vi "ConvertDataDoubleToDriveStatus.vi"(8 "error in (no error)":errorcluster, 9 "Drive Status":string(combo)="MaskValue", 10 "Double In":dbl[](array[numeric]), 11 "controller in":refnum<k24>) -> (0 "error out":errorcluster, 2 "Drive Status Out":i32[](array[numeric]), 3 "controller out":refnum<k24>)   [LabVIEW 2010]
uses:
  c:/aerotech/controller/dev/A3200/pc/labview/2010/bin/Aerotech.A3200.dll
  bin/Aerotech.A3200.dll
  c:/aerotech/controller/dev/A3200/pc/labview/2010/bin/Aerotech.A3200.LabVIEW.dll
  bin/Aerotech.A3200.LabVIEW.dll
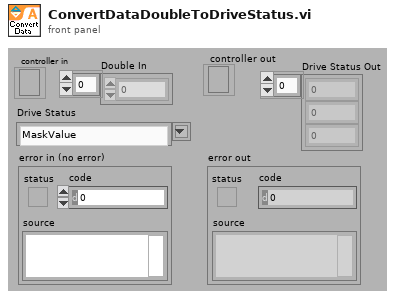
[diagram p1: front panel]
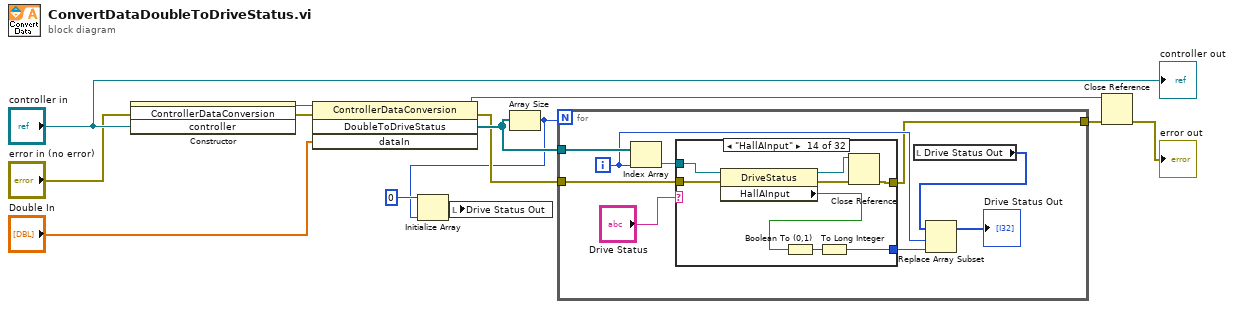
[diagram p0: block diagram]
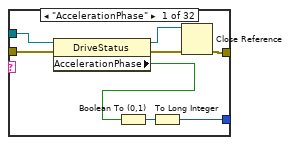
[diagram p2: hidden frame]
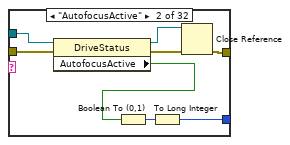
[diagram p3: hidden frame]
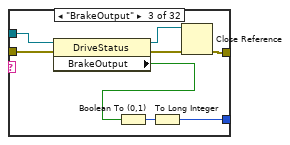
[diagram p4: hidden frame]
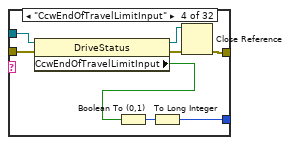
[diagram p5: hidden frame]
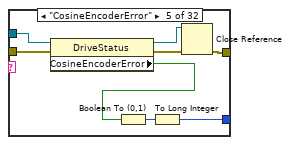
[diagram p6: hidden frame]
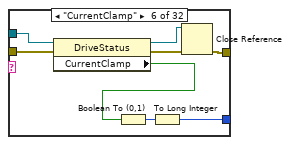
[diagram p7: hidden frame]
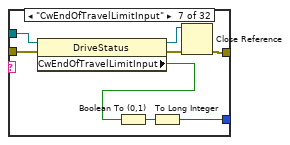
[diagram p8: hidden frame]
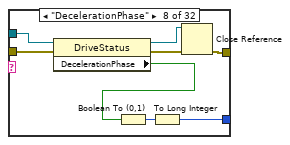
[diagram p9: hidden frame]
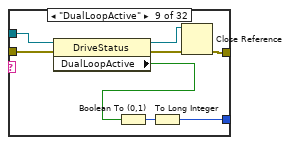
[diagram p10: hidden frame]
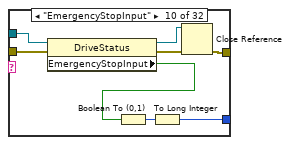
[diagram p11: hidden frame]
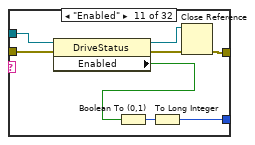
[diagram p12: hidden frame]
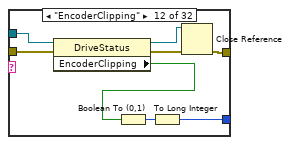
[diagram p13: hidden frame]
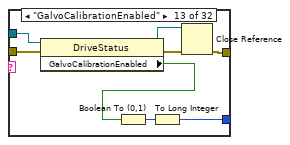
[diagram p14: hidden frame]
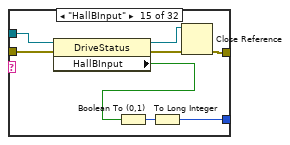
[diagram p15: hidden frame]
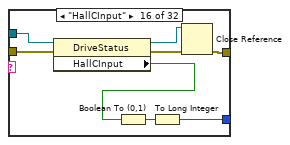
[diagram p16: hidden frame]
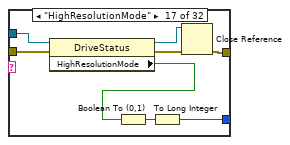
[diagram p17: hidden frame]
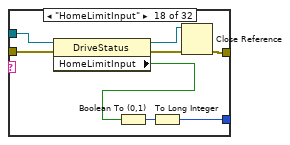
[diagram p18: hidden frame]
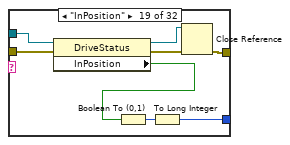
[diagram p19: hidden frame]
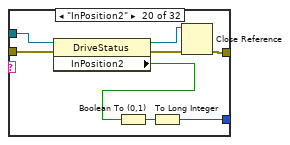
[diagram p20: hidden frame]
diagram:
  n1 = constructor class="ControllerDataConversion"(error in="error in (no error)", "controller"="controller in") -> (reference out=w13:refnum<k24>, error out=w10:errorcluster)  [unwired: 2 in, 2 out]
  n2 = invoke class="ControllerDataConversion" method="DoubleToDriveStatus"(reference=w13, error in=w10, "dataIn"="Double In") -> (reference out=w8:refnum<k24>, error out=w5:errorcluster, "DoubleToDriveStatus"=w6:refnum<k24>[])  [unwired: 1 in, 1 out]
  n3 = Array Size(array=w6) -> (size(s)=w2:i32)
  n4 = Initialize Array(0 ("element"), w2) -> (w1:i32[])
  n5 = local write "Drive Status Out"(w1) -> ()
  n6 = for {
    N: w2 -> [_]
    tunnel: w6 -> [w22]
    tunnel: w5 -> [w20]
    tunnel: [w16] -> w4
    i -> [w19]
    n7 = Index Array(array=w22, index=w19) -> (element=w21:refnum<k24>)
    n8 = case shown="\"HallAInput\"" "Drive Status" {
      tunnel: w21 -> [w30 w38 w46 w54 w62 w70 w78 w86 w94 w102 w110 w118 w126 w134 w142 w150 w158 w166 w174 w182 w190 w198 w204 w212 w220 w228 w236 w244 w252 w260 w268 w276]
      tunnel: w20 -> [w27 w35 w43 w51 w59 w67 w75 w83 w91 w99 w107 w115 w123 w131 w139 w147 w155 w163 w171 w179 w187 w195 w201 w209 w217 w225 w233 w241 w249 w257 w265 w273]
      tunnel: [w25 w33 w41 w49 w57 w65 w73 w81 w89 w97 w105 w113 w121 w129 w137 w145 w153 w161 w169 w177 w185 w193 w200 w207 w215 w223 w231 w239 w247 w255 w263 w271] -> w17
      tunnel: [w24 w32 w40 w48 w56 w64 w72 w80 w88 w96 w104 w112 w120 w128 w136 w144 w152 w160 w168 w176 w184 w192 w199 w206 w214 w222 w230 w238 w246 w254 w262 w270] -> w16
      frame "AccelerationPhase" {
        n9 = property class="DriveStatus"(reference=w30, error in=w27) -> (reference out=w29:refnum<k24>, error out=w28:errorcluster, "AccelerationPhase"=w23:bool)
        n10 = Boolean To (0,1)(Boolean=w23) -> (0, 1=w26:i16)
        n11 = To Long Integer(number=w26) -> (32bit integer=w25:i32)
        n12 = Close Reference(reference=w29, error in (no error)=w28) -> (error out=w24:errorcluster)
      }
      frame "AutofocusActive" {
        n13 = property class="DriveStatus"(reference=w38, error in=w35) -> (reference out=w37:refnum<k24>, error out=w36:errorcluster, "AutofocusActive"=w31:bool)
        n14 = Boolean To (0,1)(Boolean=w31) -> (0, 1=w34:i16)
        n15 = To Long Integer(number=w34) -> (32bit integer=w33:i32)
        n16 = Close Reference(reference=w37, error in (no error)=w36) -> (error out=w32:errorcluster)
      }
      frame "BrakeOutput" {
        n17 = property class="DriveStatus"(reference=w46, error in=w43) -> (reference out=w45:refnum<k24>, error out=w44:errorcluster, "BrakeOutput"=w39:bool)
        n18 = Boolean To (0,1)(Boolean=w39) -> (0, 1=w42:i16)
        n19 = To Long Integer(number=w42) -> (32bit integer=w41:i32)
        n20 = Close Reference(reference=w45, error in (no error)=w44) -> (error out=w40:errorcluster)
      }
      frame "CcwEndOfTravelLimitInput" {
        n21 = property class="DriveStatus"(reference=w54, error in=w51) -> (reference out=w53:refnum<k24>, error out=w52:errorcluster, "CcwEndOfTravelLimitInput"=w47:bool)
        n22 = Boolean To (0,1)(Boolean=w47) -> (0, 1=w50:i16)
        n23 = To Long Integer(number=w50) -> (32bit integer=w49:i32)
        n24 = Close Reference(reference=w53, error in (no error)=w52) -> (error out=w48:errorcluster)
      }
      frame "CosineEncoderError" {
        n25 = property class="DriveStatus"(reference=w62, error in=w59) -> (reference out=w61:refnum<k24>, error out=w60:errorcluster, "CosineEncoderError"=w55:bool)
        n26 = Boolean To (0,1)(Boolean=w55) -> (0, 1=w58:i16)
        n27 = To Long Integer(number=w58) -> (32bit integer=w57:i32)
        n28 = Close Reference(reference=w61, error in (no error)=w60) -> (error out=w56:errorcluster)
      }
      frame "CurrentClamp" {
        n29 = property class="DriveStatus"(reference=w70, error in=w67) -> (reference out=w69:refnum<k24>, error out=w68:errorcluster, "CurrentClamp"=w63:bool)
        n30 = Boolean To (0,1)(Boolean=w63) -> (0, 1=w66:i16)
        n31 = To Long Integer(number=w66) -> (32bit integer=w65:i32)
        n32 = Close Reference(reference=w69, error in (no error)=w68) -> (error out=w64:errorcluster)
      }
      frame "CwEndOfTravelLimitInput" {
        n33 = property class="DriveStatus"(reference=w78, error in=w75) -> (reference out=w77:refnum<k24>, error out=w76:errorcluster, "CwEndOfTravelLimitInput"=w71:bool)
        n34 = Boolean To (0,1)(Boolean=w71) -> (0, 1=w74:i16)
        n35 = To Long Integer(number=w74) -> (32bit integer=w73:i32)
        n36 = Close Reference(reference=w77, error in (no error)=w76) -> (error out=w72:errorcluster)
      }
      frame "DecelerationPhase" {
        n37 = property class="DriveStatus"(reference=w86, error in=w83) -> (reference out=w85:refnum<k24>, error out=w84:errorcluster, "DecelerationPhase"=w79:bool)
        n38 = Boolean To (0,1)(Boolean=w79) -> (0, 1=w82:i16)
        n39 = To Long Integer(number=w82) -> (32bit integer=w81:i32)
        n40 = Close Reference(reference=w85, error in (no error)=w84) -> (error out=w80:errorcluster)
      }
      frame "DualLoopActive" {
        n41 = property class="DriveStatus"(reference=w94, error in=w91) -> (reference out=w93:refnum<k24>, error out=w92:errorcluster, "DualLoopActive"=w87:bool)
        n42 = Boolean To (0,1)(Boolean=w87) -> (0, 1=w90:i16)
        n43 = To Long Integer(number=w90) -> (32bit integer=w89:i32)
        n44 = Close Reference(reference=w93, error in (no error)=w92) -> (error out=w88:errorcluster)
      }
      frame "EmergencyStopInput" {
        n45 = property class="DriveStatus"(reference=w102, error in=w99) -> (reference out=w101:refnum<k24>, error out=w100:errorcluster, "EmergencyStopInput"=w95:bool)
        n46 = Boolean To (0,1)(Boolean=w95) -> (0, 1=w98:i16)
        n47 = To Long Integer(number=w98) -> (32bit integer=w97:i32)
        n48 = Close Reference(reference=w101, error in (no error)=w100) -> (error out=w96:errorcluster)
      }
      frame "Enabled" {
        n49 = property class="DriveStatus"(reference=w110, error in=w107) -> (reference out=w109:refnum<k24>, error out=w108:errorcluster, "Enabled"=w103:bool)
        n50 = Boolean To (0,1)(Boolean=w103) -> (0, 1=w106:i16)
        n51 = To Long Integer(number=w106) -> (32bit integer=w105:i32)
        n52 = Close Reference(reference=w109, error in (no error)=w108) -> (error out=w104:errorcluster)
      }
      frame "EncoderClipping" {
        n53 = property class="DriveStatus"(reference=w118, error in=w115) -> (reference out=w117:refnum<k24>, error out=w116:errorcluster, "EncoderClipping"=w111:bool)
        n54 = Boolean To (0,1)(Boolean=w111) -> (0, 1=w114:i16)
        n55 = To Long Integer(number=w114) -> (32bit integer=w113:i32)
        n56 = Close Reference(reference=w117, error in (no error)=w116) -> (error out=w112:errorcluster)
      }
      frame "GalvoCalibrationEnabled" {
        n57 = property class="DriveStatus"(reference=w126, error in=w123) -> (reference out=w125:refnum<k24>, error out=w124:errorcluster, "GalvoCalibrationEnabled"=w119:bool)
        n58 = Boolean To (0,1)(Boolean=w119) -> (0, 1=w122:i16)
        n59 = To Long Integer(number=w122) -> (32bit integer=w121:i32)
        n60 = Close Reference(reference=w125, error in (no error)=w124) -> (error out=w120:errorcluster)
      }
      frame "HallAInput" {
        n61 = property class="DriveStatus"(reference=w134, error in=w131) -> (reference out=w133:refnum<k24>, error out=w132:errorcluster, "HallAInput"=w127:bool)
        n62 = Boolean To (0,1)(Boolean=w127) -> (0, 1=w130:i16)
        n63 = To Long Integer(number=w130) -> (32bit integer=w129:i32)
        n64 = Close Reference(reference=w133, error in (no error)=w132) -> (error out=w128:errorcluster)
      }
      frame "HallBInput" {
        n65 = property class="DriveStatus"(reference=w142, error in=w139) -> (reference out=w141:refnum<k24>, error out=w140:errorcluster, "HallBInput"=w135:bool)
        n66 = Boolean To (0,1)(Boolean=w135) -> (0, 1=w138:i16)
        n67 = To Long Integer(number=w138) -> (32bit integer=w137:i32)
        n68 = Close Reference(reference=w141, error in (no error)=w140) -> (error out=w136:errorcluster)
      }
      frame "HallCInput" {
        n69 = property class="DriveStatus"(reference=w150, error in=w147) -> (reference out=w149:refnum<k24>, error out=w148:errorcluster, "HallCInput"=w143:bool)
        n70 = Boolean To (0,1)(Boolean=w143) -> (0, 1=w146:i16)
        n71 = To Long Integer(number=w146) -> (32bit integer=w145:i32)
        n72 = Close Reference(reference=w149, error in (no error)=w148) -> (error out=w144:errorcluster)
      }
      frame "HighResolutionMode" {
        n73 = property class="DriveStatus"(reference=w158, error in=w155) -> (reference out=w157:refnum<k24>, error out=w156:errorcluster, "HighResolutionMode"=w151:bool)
        n74 = Boolean To (0,1)(Boolean=w151) -> (0, 1=w154:i16)
        n75 = To Long Integer(number=w154) -> (32bit integer=w153:i32)
        n76 = Close Reference(reference=w157, error in (no error)=w156) -> (error out=w152:errorcluster)
      }
      frame "HomeLimitInput" {
        n77 = property class="DriveStatus"(reference=w166, error in=w163) -> (reference out=w165:refnum<k24>, error out=w164:errorcluster, "HomeLimitInput"=w159:bool)
        n78 = Boolean To (0,1)(Boolean=w159) -> (0, 1=w162:i16)
        n79 = To Long Integer(number=w162) -> (32bit integer=w161:i32)
        n80 = Close Reference(reference=w165, error in (no error)=w164) -> (error out=w160:errorcluster)
      }
      frame "InPosition" {
        n81 = property class="DriveStatus"(reference=w174, error in=w171) -> (reference out=w173:refnum<k24>, error out=w172:errorcluster, "InPosition"=w167:bool)
        n82 = Boolean To (0,1)(Boolean=w167) -> (0, 1=w170:i16)
        n83 = To Long Integer(number=w170) -> (32bit integer=w169:i32)
        n84 = Close Reference(reference=w173, error in (no error)=w172) -> (error out=w168:errorcluster)
      }
      frame "InPosition2" {
        n85 = property class="DriveStatus"(reference=w182, error in=w179) -> (reference out=w181:refnum<k24>, error out=w180:errorcluster, "InPosition2"=w175:bool)
        n86 = Boolean To (0,1)(Boolean=w175) -> (0, 1=w178:i16)
        n87 = To Long Integer(number=w178) -> (32bit integer=w177:i32)
        n88 = Close Reference(reference=w181, error in (no error)=w180) -> (error out=w176:errorcluster)
      }
      frame "MarkerInput" {
        n89 = property class="DriveStatus"(reference=w190, error in=w187) -> (reference out=w189:refnum<k24>, error out=w188:errorcluster, "MarkerInput"=w183:bool)
        n90 = Boolean To (0,1)(Boolean=w183) -> (0, 1=w186:i16)
        n91 = To Long Integer(number=w186) -> (32bit integer=w185:i32)
        n92 = Close Reference(reference=w189, error in (no error)=w188) -> (error out=w184:errorcluster)
      }
      frame "MarkerLatch" {
        n93 = property class="DriveStatus"(reference=w198, error in=w195) -> (reference out=w197:refnum<k24>, error out=w196:errorcluster, "MarkerLatch"=w191:bool)
        n94 = Boolean To (0,1)(Boolean=w191) -> (0, 1=w194:i16)
        n95 = To Long Integer(number=w194) -> (32bit integer=w193:i32)
        n96 = Close Reference(reference=w197, error in (no error)=w196) -> (error out=w192:errorcluster)
      }
      frame "MaskValue", Default {
        n97 = property class="DriveStatus"(reference=w204, error in=w201) -> (reference out=w203:refnum<k24>, error out=w202:errorcluster, "MaskValue"=w200:i32)
        n98 = Close Reference(reference=w203, error in (no error)=w202) -> (error out=w199:errorcluster)
      }
      frame "MoveActive" {
        n99 = property class="DriveStatus"(reference=w212, error in=w209) -> (reference out=w211:refnum<k24>, error out=w210:errorcluster, "MoveActive"=w205:bool)
        n100 = Boolean To (0,1)(Boolean=w205) -> (0, 1=w208:i16)
        n101 = To Long Integer(number=w208) -> (32bit integer=w207:i32)
        n102 = Close Reference(reference=w211, error in (no error)=w210) -> (error out=w206:errorcluster)
      }
      frame "NoMotorSupply" {
        n103 = property class="DriveStatus"(reference=w220, error in=w217) -> (reference out=w219:refnum<k24>, error out=w218:errorcluster, "NoMotorSupply"=w213:bool)
        n104 = Boolean To (0,1)(Boolean=w213) -> (0, 1=w216:i16)
        n105 = To Long Integer(number=w216) -> (32bit integer=w215:i32)
        n106 = Close Reference(reference=w219, error in (no error)=w218) -> (error out=w214:errorcluster)
      }
      frame "None" {
        n107 = property class="DriveStatus"(reference=w228, error in=w225) -> (reference out=w227:refnum<k24>, error out=w226:errorcluster, "None"=w221:bool)
        n108 = Boolean To (0,1)(Boolean=w221) -> (0, 1=w224:i16)
        n109 = To Long Integer(number=w224) -> (32bit integer=w223:i32)
        n110 = Close Reference(reference=w227, error in (no error)=w226) -> (error out=w222:errorcluster)
      }
      frame "PSOHaltLatch" {
        n111 = property class="DriveStatus"(reference=w236, error in=w233) -> (reference out=w235:refnum<k24>, error out=w234:errorcluster, "PSOHaltLatch"=w229:bool)
        n112 = Boolean To (0,1)(Boolean=w229) -> (0, 1=w232:i16)
        n113 = To Long Integer(number=w232) -> (32bit integer=w231:i32)
        n114 = Close Reference(reference=w235, error in (no error)=w234) -> (error out=w230:errorcluster)
      }
      frame "PowerLimiting" {
        n115 = property class="DriveStatus"(reference=w244, error in=w241) -> (reference out=w243:refnum<k24>, error out=w242:errorcluster, "PowerLimiting"=w237:bool)
        n116 = Boolean To (0,1)(Boolean=w237) -> (0, 1=w240:i16)
        n117 = To Long Integer(number=w240) -> (32bit integer=w239:i32)
        n118 = Close Reference(reference=w243, error in (no error)=w242) -> (error out=w238:errorcluster)
      }
      frame "ProgrammingFlash" {
        n119 = property class="DriveStatus"(reference=w252, error in=w249) -> (reference out=w251:refnum<k24>, error out=w250:errorcluster, "ProgrammingFlash"=w245:bool)
        n120 = Boolean To (0,1)(Boolean=w245) -> (0, 1=w248:i16)
        n121 = To Long Integer(number=w248) -> (32bit integer=w247:i32)
        n122 = Close Reference(reference=w251, error in (no error)=w250) -> (error out=w246:errorcluster)
      }
      frame "ProgrammingMXH" {
        n123 = property class="DriveStatus"(reference=w260, error in=w257) -> (reference out=w259:refnum<k24>, error out=w258:errorcluster, "ProgrammingMXH"=w253:bool)
        n124 = Boolean To (0,1)(Boolean=w253) -> (0, 1=w256:i16)
        n125 = To Long Integer(number=w256) -> (32bit integer=w255:i32)
        n126 = Close Reference(reference=w259, error in (no error)=w258) -> (error out=w254:errorcluster)
      }
      frame "ServoControl" {
        n127 = property class="DriveStatus"(reference=w268, error in=w265) -> (reference out=w267:refnum<k24>, error out=w266:errorcluster, "ServoControl"=w261:bool)
        n128 = Boolean To (0,1)(Boolean=w261) -> (0, 1=w264:i16)
        n129 = To Long Integer(number=w264) -> (32bit integer=w263:i32)
        n130 = Close Reference(reference=w267, error in (no error)=w266) -> (error out=w262:errorcluster)
      }
      frame "SineEncoderError" {
        n131 = property class="DriveStatus"(reference=w276, error in=w273) -> (reference out=w275:refnum<k24>, error out=w274:errorcluster, "SineEncoderError"=w269:bool)
        n132 = Boolean To (0,1)(Boolean=w269) -> (0, 1=w272:i16)
        n133 = To Long Integer(number=w272) -> (32bit integer=w271:i32)
        n134 = Close Reference(reference=w275, error in (no error)=w274) -> (error out=w270:errorcluster)
      }
    }
    n135 = local read "Drive Status Out"() -> (w14:i32[])
    n136 = Replace Array Subset(array=w14, new element=w17, index=w19) -> (→"Drive Status Out":i32[])
  }
  n137 = Close Reference(reference=w8, error in (no error)=w4) -> (error out=→"error out":errorcluster)
  "controller out" <- "controller in"
